vi "ziExample-Module-MDS_Sweeper.vi"() -> ()   [LabVIEW 2009]
doc: "This examples allows to control a Zurich Instruments device via a LabOne Labview API. \nThis vi enables the multi-device synchronisation of two ZI instruments of the same family.\n\n© Zurich Instruments AG, www.zhinst.com"
uses:
  <instrlib>/Zurich Instruments LabOne/Public/Modules/ziTypeModEnum.ctl
  <instrlib>/Zurich Instruments LabOne/Public/Modules/ziModSetValueDouble.vi
  <instrlib>/Zurich Instruments LabOne/Public/Modules/ziModSetValueDoubleArray.vi
  <instrlib>/Zurich Instruments LabOne/Public/Modules/ziModSetValueBinaryArray.vi
  <instrlib>/Zurich Instruments LabOne/Public/Configure/ziSetValueDouble.vi
  <instrlib>/Zurich Instruments LabOne/Public/Modules/ziModGetSweeperData.vi
  <instrlib>/Zurich Instruments LabOne/Zurich Instruments LabOne.lvlib
panel:
  in  "Samplecount":dbl=100.0
  in  "Stop":dbl=100000.0
  in  "Start":dbl=10000.0
  in  "Gridnode":string="oscs/0/freq"
  in  "subscribepath":string="demods/0/sample" caption="Subscribe Path"
  out "Sweeper R":cluster{"grid":dbl[], "r":dbl[]}[](graph)
  out "Error Out":errorcluster
  in  "Slaves":string[](array[string])=["dev"]
  out "Status":dbl
  out "Message":string
  in  "Master":string="dev"
  # "ziExample-Module-MDS_Sweeper.vi\nRequirements: 2x(MFLI or UHF or HDAWG )\nsee block diagram for VI description"
  # "Tested Devices:\n- MFLI\n- UHF"
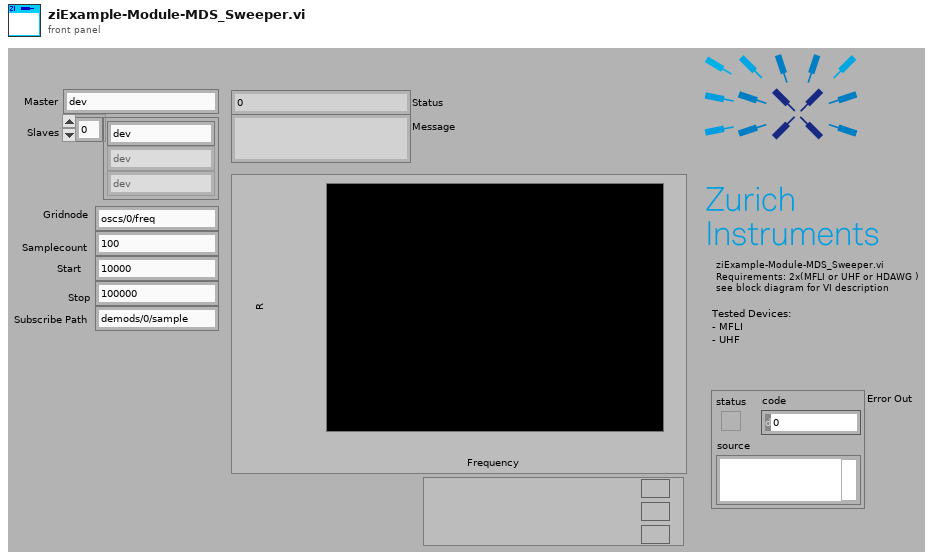
[diagram p1: front panel]
types:
  T1 = typedef "Zurich Instruments LabOne.lvlib/ziTypeModEnum.ctl" = u16
  T2 = typedef "Zurich Instruments LabOne.lvlib/ziTypeHandle.ctl" = cluster{"handleValid":bool, "Conn":u64, "Path Prefix":string, "Handle":u64, "Connected":bool, "Clockbase(s)":dbl}
  T3 = typedef "Zurich Instruments LabOne.lvlib/ziTypeModHandle.ctl" = cluster{"handleValid":bool, "Conn":u64, "ModHandle":u64, "moduleID":string, "Path Prefix":string}
  T4 = typedef "Zurich Instruments LabOne.lvlib/ziTypeModResults.ctl" = cluster{"PathArray":string[], "ValueType":T5, "NoOfResults":u64, "ziGenericHeader":T6[]}
  T5 = typedef "Zurich Instruments LabOne.lvlib/ziTypePollType.ctl" = enum16{"NONE", "DOUBLE_DATA", "INTEGER_DATA", "DEMOD_SAMPLE", "SCOPE_WAVE_HF2", "AUXIN_SAMPLE", "DIO_SAMPLE", "BYTE_ARRAY", "PWA_WAVE", "9", "10", "11", "12", "13", "14", "15", "TREE_CHANGE_DEPRI", "17", "ERROR", "19", "20", "21", "22", "23", "24", "25", "26", "27", "28", "29", "30", "31", "DOUBLE_DATA_TS", "INTEGER_DATA_TS", "34", "SCOPE_WAVE", "SCOPE_WAVE_EX", "37", "BYTE_ARRAY_TS", "39", "40", "41", "42", "43", "44", "45", "CNT_DATA", "47", "TREE_CHANGE", "49", "50", "51", "52", "53", "54", "55", "56", "57", "58", "59", "60", "61", "62", "63", "SWEEPER_DATA", "SPECTRUM_DATA", "ADVISOR_DATA", "VECTOR_DATA", "IMP_DATA"}
  T6 = typedef "Zurich Instruments LabOne.lvlib/ziTypeModGenericHeader.ctl" = cluster{"HeaderType":enum8{"HEADER_TYPE_NONE", "HEADER_TYPE_SWTRIGGER", "HEADER_TYPE_SWEEPER"}, "SampleFormat":u8, "SystemTime":timestamp, "CreatedTimeStamp":u64, "ChangedTimeStamp":u64, "Flags":u32, "ChunkSizeBytes":u64, "Name":string, "Status":u32, "GroupIndex":u32, "Color":u32, "ActiveRow":u32, "TriggerNumber":u64, "GridRows":u32, "GridCols":u32, "GridMode":u32, "GridOperation":u32, "GridDirection":u32, "GridRepetitions":u32, "GridColDelta":dbl, "GridColOffset":dbl, "GridRowDelta":dbl, "GridRowOffset":dbl, "Bandwidth":dbl, "Center":dbl, "Nenbw":dbl}
  T7 = typedef "Zurich Instruments LabOne.lvlib/ziTypeModSweeperDemodWave.ctl" = cluster{"timestamp":u64, "sampleCount":u64, "flags":u8, "sampleFormat":u8, "sweepMode":u8, "bandwidthMode":u8, "count":u64[], "settimestamp":u64[], "nexttimestamp":u64[], "grid":dbl[], "bandwidth":dbl[], "tc":dbl[], "tcmeas":dbl[], "settling":dbl[], "x":dbl[], "xstddev":dbl[], "xpwr":dbl[], "y":dbl[], "ystddev":dbl[], "ypwr":dbl[], "r":dbl[], "rstddev":dbl[], "rpwr":dbl[], "phase":dbl[], "phasestddev":dbl[], "phasepwr":dbl[], "frequency":dbl[], "frequencystddev":dbl[], "frequencypwr":dbl[], "auxin0":dbl[], "auxin0stddev":dbl[], "auxin0pwr":dbl[], "auxin1":dbl[], "auxin1stddev":dbl[], "auxin1pwr":dbl[]}
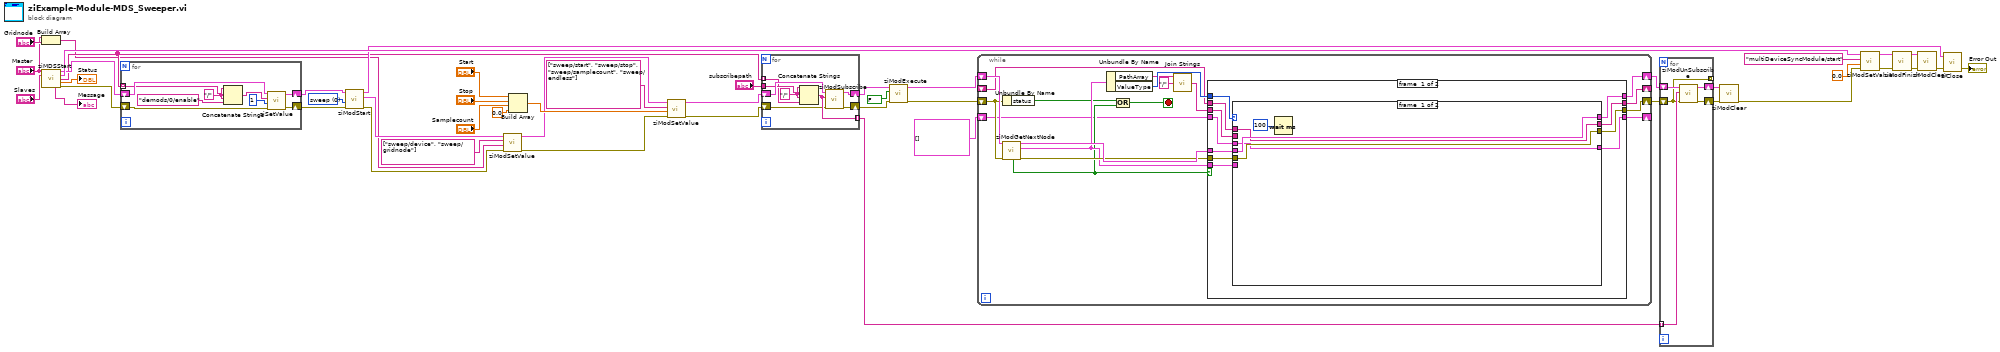
[diagram p0: block diagram]
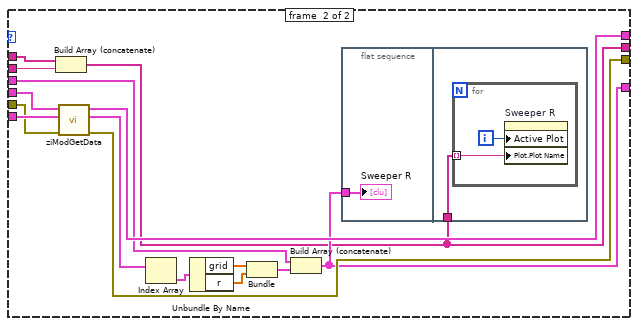
[diagram p2: hidden frame]
diagram:
  w25 = T1 0 items=["sweep", "scopeModule", "dataAcquisitionModule", "pidAdvisor", "awgModule", "impedanceModule", "multiDeviceSyncModule", "zoomFFT", "trigger", "deviceSettings", "record"] ("module Id")
  n1 = Build Array("Master", "Gridnode") -> (w3:string[])
  n2 = call <instrlib>:"ziMDSStart.vi"("Master"="Master", "Slaves"="Slaves") -> ("Handle Out"=w15:T2, "ModHandle Out"=w41:T3, "MDS_Devices"=w13:string[], "Status"=→"Status":dbl, "Message"=→"Message":string, "Error Out"=w14:errorcluster)  [unwired: 8 in]
  n3 = for {
    shift-right: [w56] -> w12
    shift-left: w14 -> [w54]
    shift-right: [w55] -> w11
    shift-left: w15 -> [w53]
    tunnel: w13 -> [w49] mode=indexing
    w57 = "/" ("string")
    n4 = Concatenate Strings(w57, w49, w57, "demods/0/enable") -> (w51:string)
    n5 = call-poly <instrlib>:"ziSetValue.vi"("Error In"=w54, "Value"=1, "Path"=w51, "Handle In"=w53) -> ("Error Out"=w56:errorcluster, "Handle Out"=w55:T2)  [unwired: 1 in]
  }
  n6 = call <instrlib>:"ziModStart.vi"("Error In"=w12, "module Id"=w25, "Handle In"=w11) -> ("Error Out"=w31:errorcluster, "ModHandle Out"=w32:T3, "Handle Out"=w24:T2)  [unwired: 6 in]
  n7 = call-poly <instrlib>:"ziModSetValue.vi"("Error In"=w31, "Values"=w3, "Paths"=string[] ["sweep/device", "sweep/gridnode"], "ModHandle In"=w32) -> ("Error Out"=w2:errorcluster, "ModHandle Out"=w1:T3)  [unwired: 6 in]
  n8 = Build Array("Start", "Stop", "Samplecount", 0.0 ("element")) -> (w26:dbl[])
  n9 = call-poly <instrlib>:"ziModSetValue.vi"("Error In"=w2, "Values"=w26, "Paths"=string[] ["sweep/start", "sweep/stop", "sweep/samplecount", "sweep/endless"], "ModHandle In"=w1) -> ("Error Out"=w20:errorcluster, "ModHandle Out"=w21:T3)  [unwired: 6 in]
  n10 = for {
    tunnel: "subscribepath" -> [w60]
    tunnel: w13 -> [w62] mode=indexing
    shift-right: [w64] -> w7
    shift-left: w20 -> [w58]
    shift-right: [w65] -> w8
    shift-left: w21 -> [w63]
    tunnel: [w59] -> w22 mode=indexing
    w61 = "/" ("string")
    n11 = Concatenate Strings(w61, w62, w61, w60) -> (w59:string)
    n12 = call <instrlib>:"ziModSubscribe.vi"("Error In"=w58, "Path"=w59, "ModHandle In"=w63) -> ("Error Out"=w64:errorcluster, "ModHandle Out"=w65:T3)  [unwired: 6 in]
  }
  n13 = call <instrlib>:"ziModExecute.vi"("Error In"=w7, "Modal (F)"=FALSE ("Modal"), "ziModHandle In"=w8) -> ("Error Out"=w33:errorcluster, "ziModHandle Out"=w35:T3)  [unwired: 5 in, 1 out]
  n14 = while {
    shift-right: [w81] -> w16
    shift-left: w35 -> [w83]
    shift-right: [w73] -> w17
    shift-left: w33 -> [w76]
    shift-right: [w71] -> _
    shift-left: cluster{"grid":dbl[], "r":dbl[]}[] [] -> [w72]
    shift-right: [w69] -> _
    shift-left: _ -> [w70]
    stop <- w75 stop-if-true
    n15 = Unbundle By Name(w76) -> ("status"=w77:bool)
    n16 = call <instrlib>:"ziModGetNextNode.vi"("Error In"=w76, "ModHandle In"=w83) -> ("Error Out"=w80:errorcluster, "ModResults"=w78:T4, "ModHandle Out"=w82:T3, "NoData"=w74:bool)  [unwired: 6 in]
    n17 = Unbundle By Name(w78) -> ("PathArray"=w68:string[], "ValueType"=w79:T5)
    n18 = Or(x=w77, y=w74) -> (x .or. y?=w75:bool)
    n19 = call <vilib>:"Join Strings.vi"("Separator (,)"="/", "Strings In"=w68) -> ("String"=w66:string)  [unwired: 1 in]
    n20 = case shown="False" w74 {
      tunnel: w82 -> [w94 w121]
      tunnel: [w93 w121] -> w81
      tunnel: [w92 w122] -> w73
      tunnel: w80 -> [w91 w122]
      tunnel: w78 -> [w90 _]
      tunnel: w79 -> [w89 _]
      tunnel: w72 -> [w88 w120]
      tunnel: [w87 w120] -> w71
      tunnel: w66 -> [w86 _]
      tunnel: [w85 w119] -> w69
      tunnel: w70 -> [w84 w119]
      frame #0 {
        n21 = case shown="\"SWEEPER_DATA\"" w89 {
          tunnel: w94 -> [w99 w107]
          tunnel: w90 -> [_ w114]
          tunnel: w91 -> [w98 w113]
          tunnel: [w98 w112] -> w92
          tunnel: [w99 w111] -> w93
          tunnel: w88 -> [w96 w105]
          tunnel: [w96 w101] -> w87
          tunnel: w86 -> [_ w103]
          tunnel: [w95 w100] -> w85
          tunnel: w84 -> [w95 w102]
          frame #0 {
            n22 = Wait (ms)(milliseconds to wait=u32 100) -> ()  [unwired: 1 out]
          }
          frame #1 {
            n23 = Build Array (concatenate)(w102, w103) -> (w100:string[])
            n24 = call-poly <instrlib>:"ziModGetData.vi"("Error In"=w113, "ModResults"=w114, "ModHandle In"=w107) -> ("Error Out"=w112:errorcluster, "SweeperDemodWaveArray"=w106:T7[], "ModHandle Out"=w111:T3)  [unwired: 4 in, 2 out]
            n25 = Index Array(array=w106) -> (element=w108:T7)  [unwired: 1 in]
            n26 = Unbundle By Name(w108) -> ("grid"=w109:dbl[], "r"=w110:dbl[])
            n27 = Bundle("grid"=w109, "r"=w110) -> (w104:cluster{"grid":dbl[], "r":dbl[]})  [unwired: 1 in]
            n28 = Build Array (concatenate)(w105, w104) -> (w101:cluster{"grid":dbl[], "r":dbl[]}[])
            n29 = flat-sequence {
              tunnel: w101 -> [w115]
              tunnel: w100 -> [w116]
              frame #0 {
                "Sweeper R" <- w115
              }
              frame #1 {
                n30 = for {
                  tunnel: w116 -> [w117] mode=indexing
                  i -> [w118]
                  n31 = property on="Sweeper R" class="XYGraph (strict)"("Active Plot"=w118, "Plot.Plot Name"=w117) -> ()  [unwired: 2 in, 2 out]
                }
              }
            }
          }
        }
      }
      frame #1 {
      }
    }
  }
  n32 = for {
    tunnel: w22 -> [w124] mode=indexing
    shift-right: [w126] -> w19
    shift-left: w16 -> [w125]
    shift-right: [w127] -> w18
    shift-left: w17 -> [w123]
    tunnel: [w123] -> _ mode=indexing
    n33 = call <instrlib>:"ziModUnSubscribe.vi"("Error In"=w123, "Path (\"/\")"=w124, "ModHandle In"=w125) -> ("Error Out"=w127:errorcluster, "ModHandle Out"=w126:T3)  [unwired: 7 in]
  }
  n34 = call <instrlib>:"ziModClear.vi"("Error In"=w18, "ziModHandle In"=w19) -> ("Error Out"=w38:errorcluster)  [unwired: 7 in, 1 out]
  n35 = call-poly <instrlib>:"ziModSetValue.vi"("Error In"=w38, "Value"=0.0, "Path"="multiDeviceSyncModule/start", "ModHandle In"=w41) -> ("Error Out"=w37:errorcluster, "ModHandle Out"=w40:T3)  [unwired: 6 in]
  n36 = call <instrlib>:"ziModFinish.vi"("Error In"=w37, "ziModHandle In"=w40) -> ("Error Out"=w48:errorcluster, "ziModHandle Out"=w47:T3)  [unwired: 7 in]
  n37 = call <instrlib>:"ziModClear.vi"("Error In"=w48, "ziModHandle In"=w47) -> ("Error Out"=w43:errorcluster)  [unwired: 7 in, 1 out]
  n38 = call <instrlib>:"ziClose.vi"("Error In"=w43, "Handle In"=w24) -> ("Error Out"=→"Error Out":errorcluster)  [unwired: 2 in, 1 out]
